vi "Utility_Read_Mixture_XML.vi"(11 "path":string) -> (3 "xmlout":string)   [LabVIEW 2015]
doc: "Reads pure fluid names from files in a given directory."
panel:
  out "Pre-defined Mixtures in REFPROP":string[][](table)=[["Air", "NITROGEN (78.12%), ARGON (0.92%), OXYGEN (20.96%)"], ["R401A", "R22 (57.89%), R152A (18.59%), R124 (23.53%)"], ["R401B", "R22 (65.49%), R152A (15.46%), R124 (19.05%)"], ["R401C", "R22 (38.56%), R152A (22.94%), R124 (38.50%)"], ["R402A", "R125 (50.77%), PROPANE (4.61%), R22 (44.63%)"], ["R402B", "R125 (29.99%), PROPANE (4.30%), R22 (65.72%)"], ["R403A", "PROPANE (10.43%), R22 (79.79%), R218 (9.78%)"], ["R403B", "PROPANE (11.71%), R22 (66.87%), R218 (21.42%)"], ["R404A", "R125 (35.78%), R134A (3.83%), R143A (60.39%)"], ["R405A", "R22 (58.24%), R152A (11.86%), R142B (6.12%), RC318 (23.78%)"], ["R406A", "R22 (57.16%), ISOBUTAN (6.18%), R142B (36.66%)"], ["R407A", "R32 (34.64%), R125 (30.03%), R134A (35.33%)"], ["R407B", "R32 (19.79%), R125 (60.04%), R134A (20.18%)"], ["R407C", "R32 (38.11%), R125 (17.96%), R134A (43.93%)"], ["R407D", "R32 (26.23%), R125 (11.37%), R134A (62.41%)"], ["R407E", "R32 (40.26%), R125 (10.47%), R134A (49.27%)"], ["R408A", "R125 (5.07%), R143A (47.63%), R22 (47.30%)"], ["R409A", "R22 (67.61%), R124 (17.85%), R142B (14.54%)"], ["R409B", "R22 (72.67%), R124 (17.71%), R142B (9.62%)"], ["R410A", "R32 (69.76%), R125 (30.24%)"], ["R410B", "R32 (65.37%), R125 (34.63%)"], ["R411A", "PROPYLEN (2.94%), R22 (83.35%), R152A (13.72%)"], ["R411B", "PROPYLEN (5.92%), R22 (90.30%), R152A (3.77%)"], ["R412A", "R22 (74.62%), R218 (2.45%), R142B (22.93%)"], ["R413A", "R218 (4.98%), R134A (89.66%), ISOBUTAN (5.37%)"], ["R414A", "R22 (57.17%), R124 (20.24%), ISOBUTAN (6.67%), R142B (15.92%)"], ["R414B", "R22 (58.74%), R124 (29.03%), ISOBUTAN (2.62%), R142B (9.60%)"], ["R415A", "R22 (77.68%), R152A (22.32%)"], ["R415B", "R22 (20.29%), R152A (79.71%)"], ["R416A", "R134A (64.72%), R124 (32.39%), BUTANE (2.89%)"], ["R417A", "R125 (41.45%), R134A (52.31%), BUTANE (6.24%)"], ["R418A", "PROPANE (2.88%), R22 (93.92%), R152A (3.20%)"], ["R419A", "R125 (70.15%), R134A (20.36%), DME (9.49%)"], ["R420A", "R134A (87.84%), R142B (12.16%)"], ["R421A", "R125 (54.00%), R134A (46.00%)"], ["R421B", "R125 (82.81%), R134A (17.19%)"], ["R422A", "R125 (80.55%), R134A (12.80%), ISOBUTAN (6.65%)"], ["R422B", "R125 (49.73%), R134A (44.67%), ISOBUTAN (5.60%)"], ["R422C", "R125 (77.48%), R134A (16.67%), ISOBUTAN (5.85%)"], ["R422D", "R125 (59.63%), R134A (33.94%), ISOBUTAN (6.43%)"], ["R423A", "R134A (64.81%), R227EA (35.19%)"], ["R424A", "R125 (45.62%), R134A (49.94%), ISOBUTAN (1.68%), BUTANE (1.87%), IPENTANE (0.90%)"], ["R425A", "R32 (32.11%), R134A (61.51%), R227EA (6.37%)"], ["R426A", "R125 (4.32%), R134A (92.57%), BUTANE (2.27%), IPENTANE (0.84%)"], ["R427A", "R32 (26.08%), R125 (18.84%), R143A (10.76%), R134A (44.32%)"], ["R428A", "R125 (69.43%), R143A (25.59%), PROPANE (1.46%), ISOBUTAN (3.52%)"], ["R500", "R12 (60.61%), R152A (39.39%)"], ["R501", "R22 (80.75%), R12 (19.25%)"], ["R502", "R22 (63.00%), R115 (37.00%)"], ["R503", "R23 (49.97%), R13 (50.03%)"], ["R504", "R32 (73.42%), R115 (26.58%)"], ["R507A", "R125 (41.18%), R143A (58.82%)"], ["R508A", "R23 (55.76%), R116 (44.24%)"], ["R508B", "R23 (62.68%), R116 (37.32%)"], ["R509A", "R22 (63.08%), R218 (36.92%)"]]
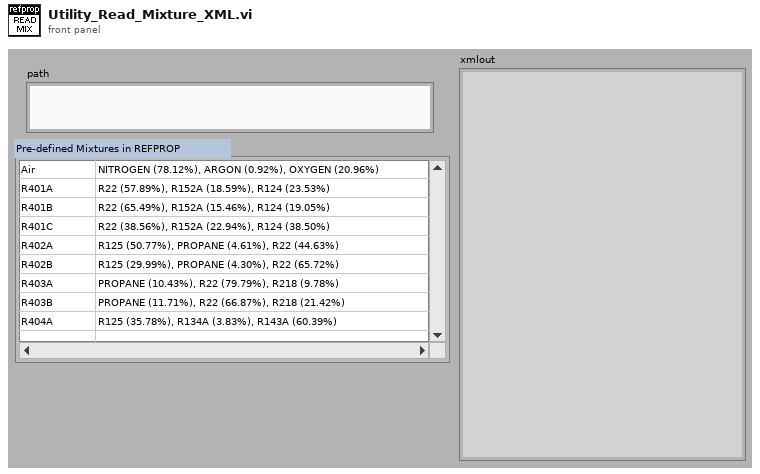
[diagram p1: front panel]
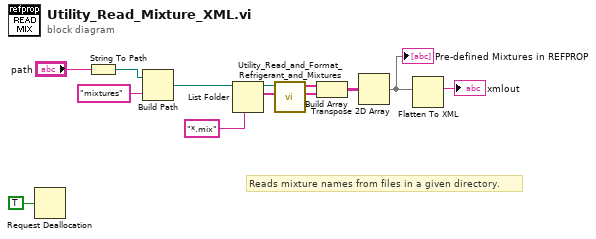
[diagram p0: block diagram]
diagram:
  # "Reads mixture names from files in a given directory."
  n1 = Request Deallocation(TRUE ("标志")) -> ()
  n2 = String To Path(string="path") -> (path=w2:path)
  n3 = Build Path(base path=w2, name or relative path="mixtures") -> (appended path=w11:path)
  n4 = List Folder(path=w11, pattern="*.mix") -> (path out=w10:path, filenames=w9:string[])  [unwired: 2 in, 2 out]
  n5 = call "Utility_Read_and_Format_Refrigerant_and_Mixtures.vi"("File names"=w9, "Refprop Fluid or Mixture Directory"=w10) -> ("Refrigerant/Mixture Info"=w6:string[], "Refrigerant/Mixture Name"=w7:string[])  [unwired: 5 in, 1 out]
  n6 = Build Array(w7, w6) -> (w8:string[][])
  n7 = Transpose 2D Array(2D array=w8) -> (transposed array=w3:string[][])
  "Pre-defined Mixtures in REFPROP" <- w3
  n8 = Flatten To XML(anything=w3) -> (xml string=→"xmlout":string)
